vi "Main.vi"(11 "Module Admin":refnum<class "Delacor_lib_QMH_Module Admin.lvclass">) -> ()   [LabVIEW 2024, in "MoneyControl.lvlib"]
doc: "This template is based off of the Queued Message Handler design pattern and the Queued Message Handler project template that ships with LabVIEW.\n\nThe main difference is that the queue is private to this module and communication between modules is performed via Broadcast and Request events.\n\nRequest events are wrapped in public API methods and are handled in the Event Handling Loop (EHL) of this VI. Any module can register for Broadcast events sent by this module. The EHL generates messages based on user interface actions.\n\nThe Message Handling Loop (MHL) processes messages generated by the EHL, or by other messages. The messages are string values, so new messages can be added easily to the Message Cases case structure in the MHL. Each message cluster can also provide an optional value for Message Data, which is a variant that can be converted to whatever message-specific data is required.\n_____\nBased on DQMH Dev Tools: Project Template 7.1.0.1503."
uses:
  MoneyControl.lvlib
  <vilib>/Delacor/Delacor QMH/Libraries/Module Admin_class/Delacor_lib_QMH_Module Admin.lvclass
  Module Data--cluster.ctl
  Stop Argument--cluster.ctl
  <vilib>/Delacor/Delacor QMH/Libraries/Message Queue_class/Delacor_lib_QMH_Message Queue.lvclass/Delacor_lib_QMH_Message Queue.ctl
  <vilib>/Delacor/Delacor QMH/Libraries/Module Admin_class/Delacor_lib_QMH_Module Admin.lvclass/Delacor_lib_QMH_Module Admin.ctl
  Draw FP in Subpanel Argument--cluster.ctl
  Remove From Subpanel Argument--cluster.ctl
  Incrementar Credito Argument--cluster.ctl
  Cancelar Argument--cluster.ctl
  <vilib>/Utility/miscctls.llb/LVFontTypeDef.ctl
  Regresa Cambio Argument--cluster.ctl
  <vilib>/Delacor/Delacor QMH/Libraries/Message Queue_class/Delacor_lib_QMH_Enqueue Message (Single).vi
  <vilib>/Delacor/Delacor QMH/Libraries/Module Admin_class/Delacor_lib_QMH_Get External Launch.vi
  63c2000c-1515-4b81-a1f2-5954ab6849f9.vi
  <vilib>/Delacor/Delacor QMH/Libraries/Message Queue_class/Delacor_lib_QMH_Message Queue.lvclass
  <vilib>/PantherLAB/Message Module/Libraries/Message/PantherLAB_lib_Message.lvlib
panel:
  in  "0.20":bool
  out "Status":string
  in  "1":bool
  in  "0.50":bool
  in  "2":bool
  out "error out":errorcluster
  in  "Cancelar":bool
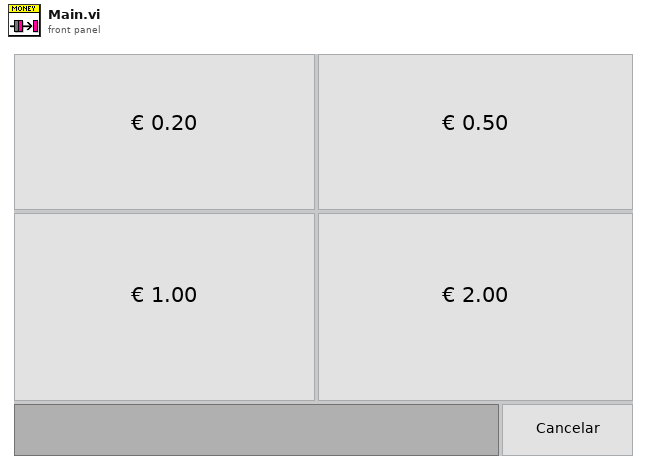
[diagram p1: front panel]
types:
  T1 = typedef "MoneyControl.lvlib/Request Events--cluster.ctl" = cluster{"Stop Module":refnum<user-event>, "Show Panel":refnum<user-event>, "Hide Panel":refnum<user-event>, "Get Module Execution Status":refnum<user-event>, "Show Diagram":refnum<user-event>, "Draw FP in Subpanel":refnum<user-event>, "Remove From Subpanel":refnum<user-event>, "Incrementar Credito":refnum<user-event>, "Cancelar":refnum<user-event>, "Regresa Cambio":refnum<user-event>}
  T2 = typedef "PantherLAB_lib_Message.lvlib/Broadcast Events--cluster.ctl" = cluster{"Module Did Init":refnum<user-event>, "Status Updated":refnum<user-event>, "Error Reported":refnum<user-event>, "Module Did Stop":refnum<user-event>, "Update Module Execution Status":refnum<user-event>}
  T3 = typedef "MoneyControl.lvlib/Module Data--cluster.ctl" = cluster{"Status":string, "Sub Panel":refnum<vi>, "Credito":dbl}
  T4 = enum32{"invalid lock state", "Not Locked", "Locked (No Password)", "Password-protected"}
  T5 = typedef "MoneyControl.lvlib/Stop Argument--cluster.ctl" = cluster{"Origin":string, "Exit via Stop Module Req?":bool, "Wait for Module to stop?":bool}
  T6 = typedef "MoneyControl.lvlib/Draw FP in Subpanel Argument--cluster.ctl" = cluster{"Sub Panel":refnum<vi>}
  T7 = typedef "MoneyControl.lvlib/Remove From Subpanel Argument--cluster.ctl" = cluster{"Boolean":bool}
  T8 = typedef "MoneyControl.lvlib/Incrementar Credito Argument--cluster.ctl" = cluster{"Dinero":dbl}
  T9 = typedef "MoneyControl.lvlib/Cancelar Argument--cluster.ctl" = cluster{"Boolean":bool}
  T10 = typedef "LVFontTypeDef.ctl" = cluster{"Font Name":string, "Size":u16, "Bold":bool, "Italic":bool, "Underline":bool, "Strikeout":bool, "Color":u32}
  T11 = typedef "MoneyControl.lvlib/Regresa Cambio Argument--cluster.ctl" = cluster{"Costo de Producto Vendido":dbl}
  T12 = enum32{"Invalid", "Standard", "Closed", "Hidden", "Minimized", "Maximized"}
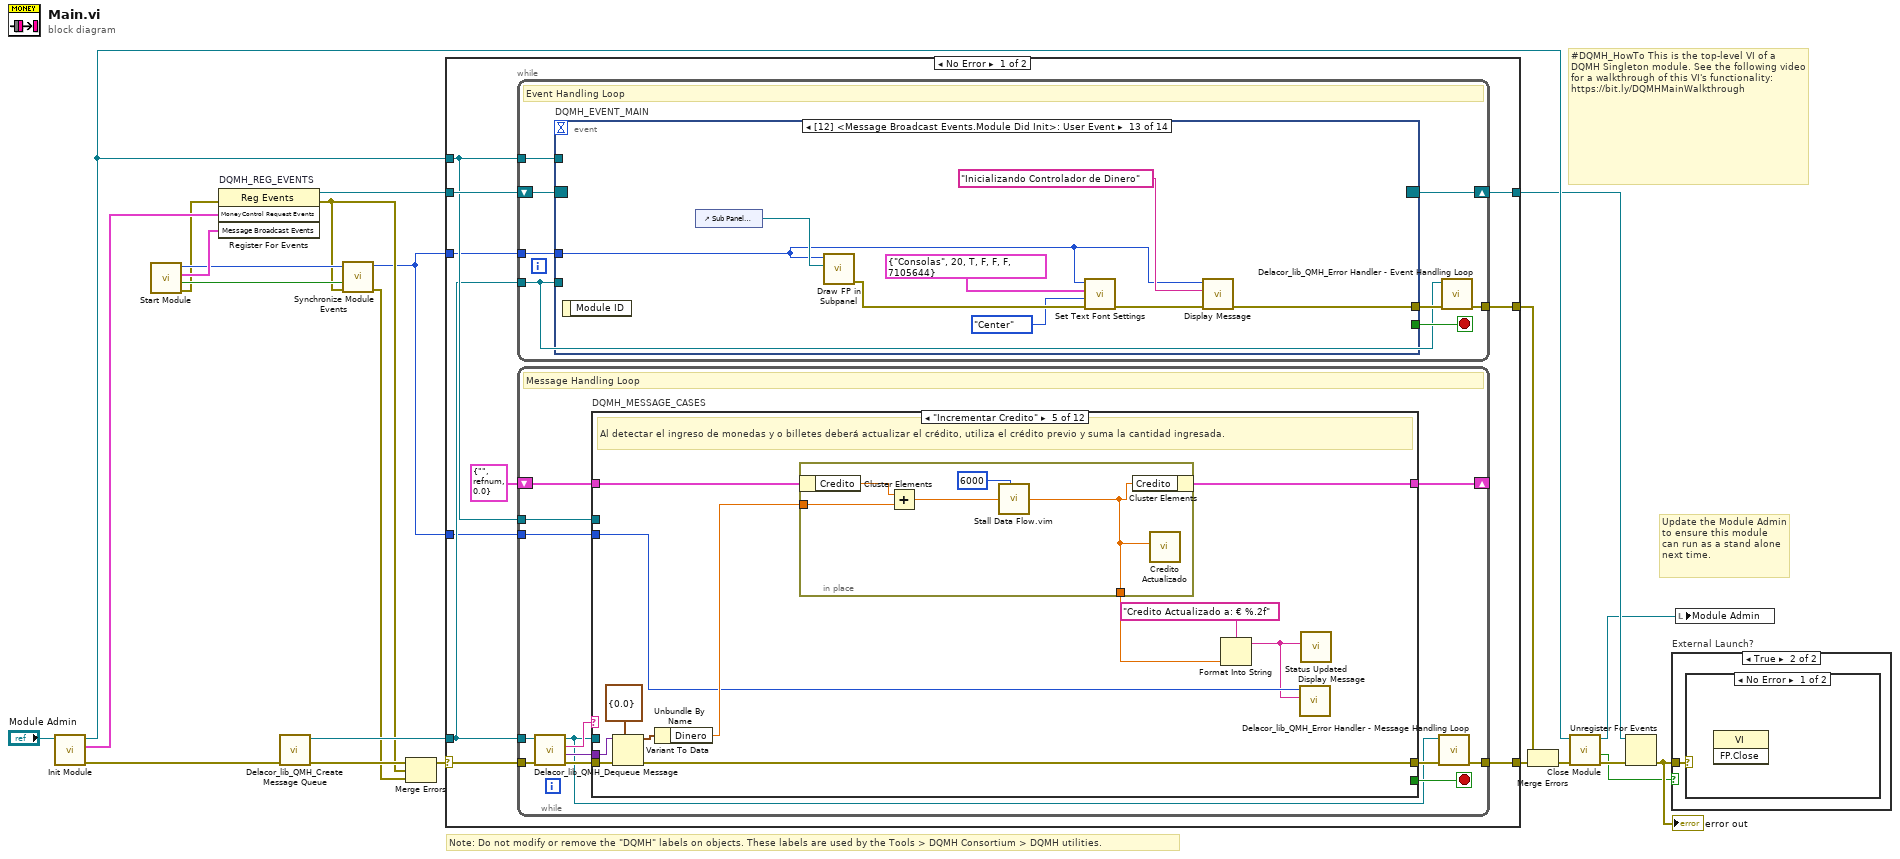
[diagram p0: block diagram]
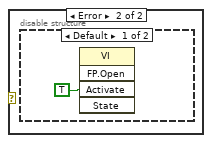
[diagram p3: hidden frame]
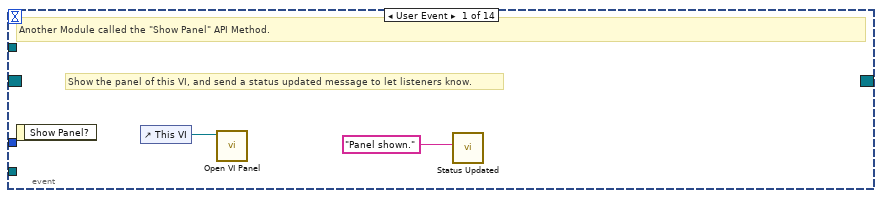
[diagram p5: hidden frame]
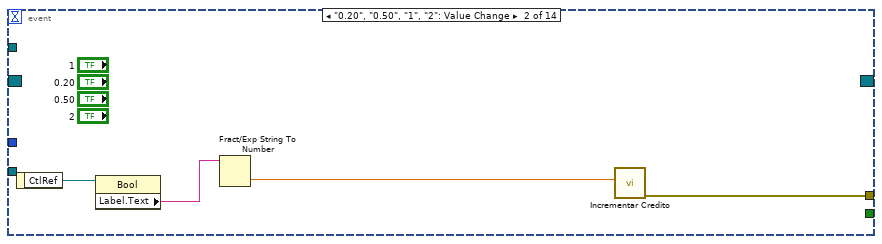
[diagram p6: hidden frame]
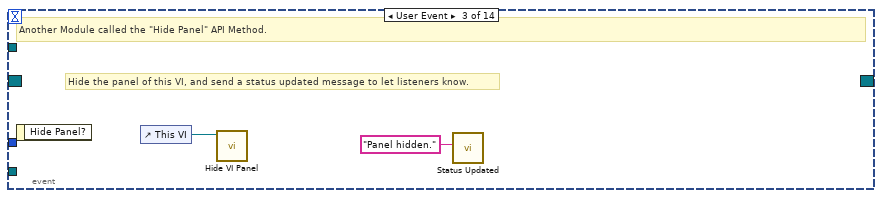
[diagram p7: hidden frame]
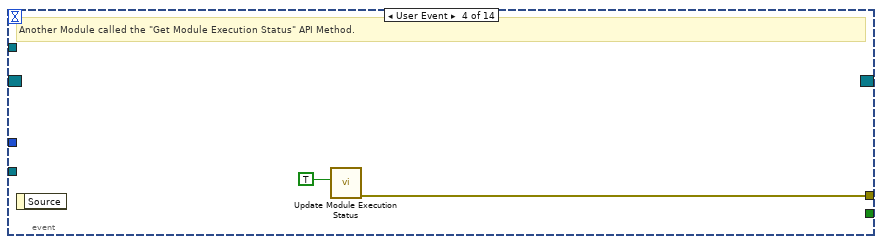
[diagram p8: hidden frame]
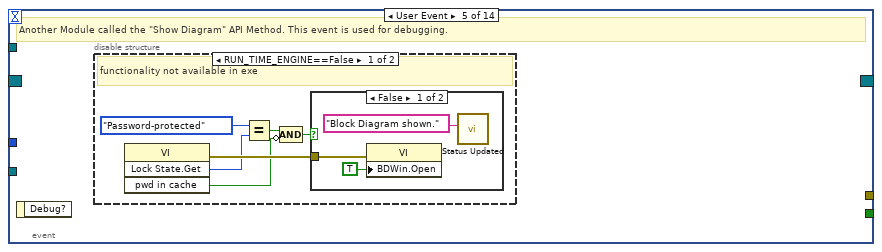
[diagram p9: hidden frame]
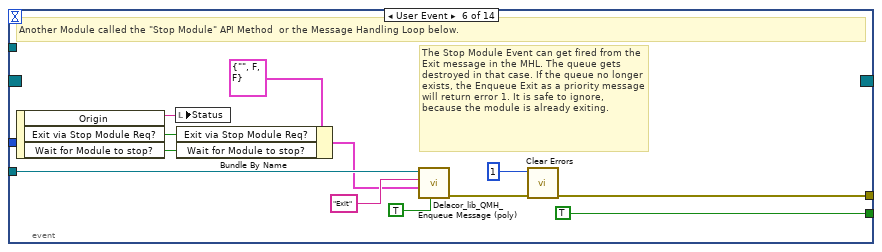
[diagram p12: hidden frame]
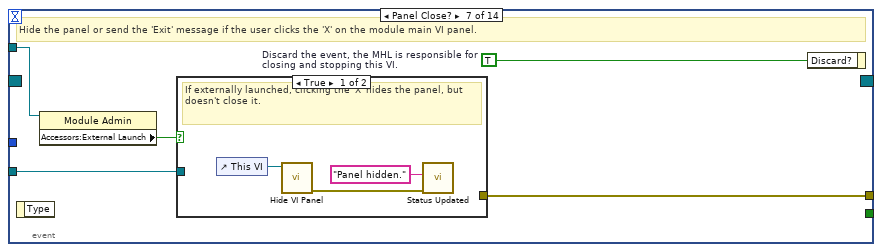
[diagram p13: hidden frame]
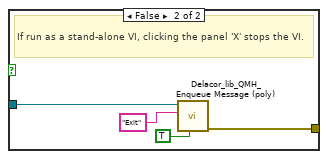
[diagram p14: hidden frame]
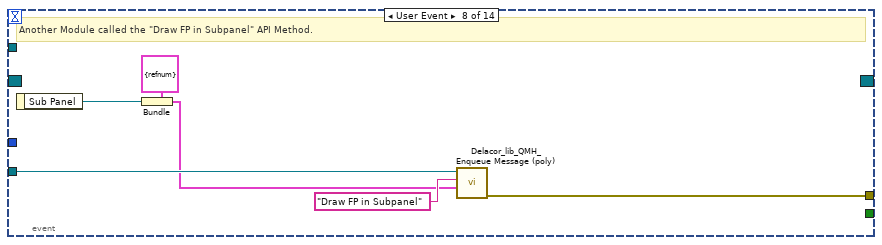
[diagram p15: hidden frame]
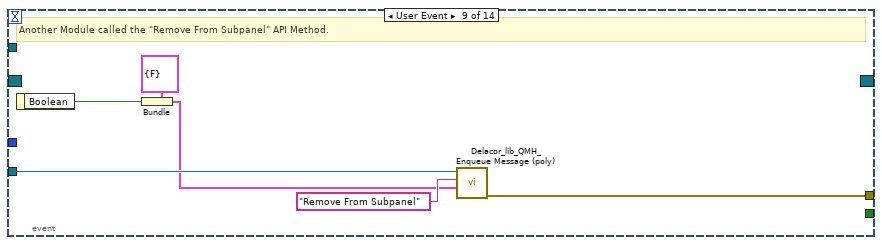
[diagram p16: hidden frame]
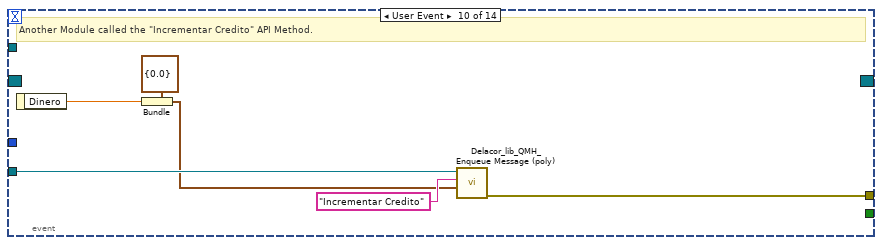
[diagram p17: hidden frame]
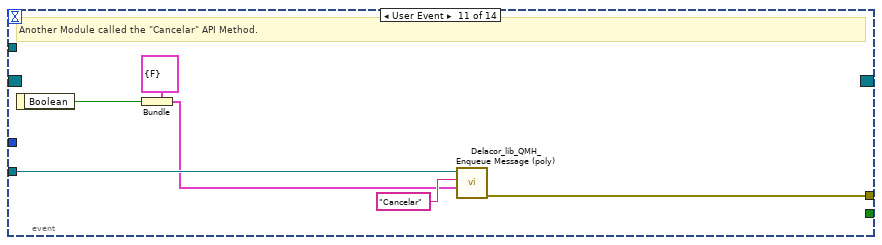
[diagram p18: hidden frame]
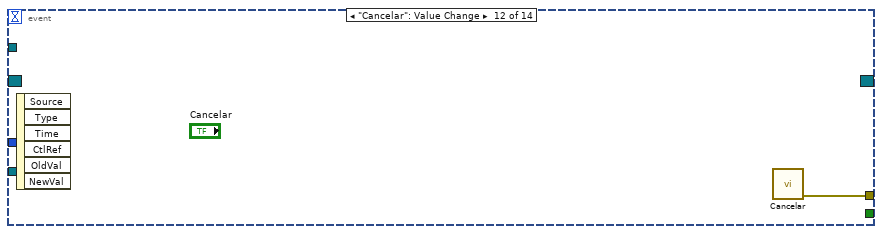
[diagram p19: hidden frame]
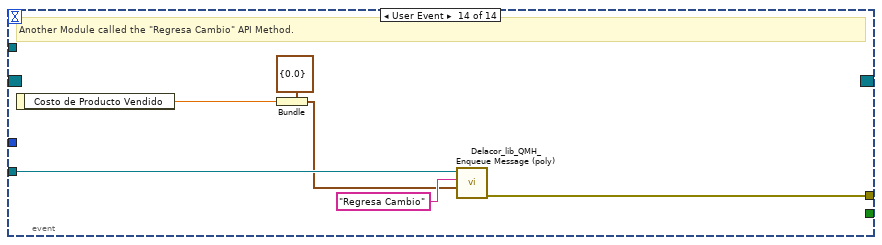
[diagram p20: hidden frame]
diagram:
  # "#DQMH_HowTo This is the top-level VI of a DQMH Singleton module. See the following video for a walkthrough of this VI's functionality: https://bit.ly/DQMHMainWalkthrough"
  # "Note: Do not modify or remove the \"DQMH\" labels on objects. These labels are used by the Tools > DQMH Consortium > DQMH utilities."
  # "Update the Module Admin to ensure this module can run as a stand alone next time."
  n1 = call "Init Module.vi"("Singleton Module Admin in"="Module Admin") -> ("error out"=w22:errorcluster, "MoneyControl Request Events"=w12:T1, "Singleton Module Admin out"=w15:refnum<class "Delacor_lib_QMH_Module Admin.lvclass">)  [unwired: 8 in]
  n2 = call <vilib>:"Start Module.vi"() -> ("error out"=w4:errorcluster, "Wait for Event Sync?"=w5:bool, "Message Broadcast Events"=w7:T2, "Module ID"=w6:i32)  [unwired: 7 in, 1 out]
  n3 = register-events "DQMH_REG_EVENTS"(error in=w4, w12, w7) -> (reference out=w13:refnum<event-registration>, error out=w3:errorcluster)  [unwired: 1 in]
  n4 = call <vilib>:"Delacor_lib_QMH_Create Message Queue.vi"("error in"=w22) -> ("error out"=w17:errorcluster, "Message Queue"=w11:refnum<class "Delacor_lib_QMH_Message Queue.lvclass">)  [unwired: 9 in]
  n5 = call <vilib>:"Synchronize Module Events.vi"("error in"=w3, "Wait for Event Sync?"=w5, "Module ID in"=w6) -> ("error out"=w2:errorcluster, "Module ID out"=w1:i32)  [unwired: 7 in]
  n6 = Merge Errors(w17, w3, w2) -> (w16:errorcluster)
  n7 = case shown="No Error" w16 {
    selector: w16 -> [w31 w304]
    tunnel: [w33 w303] -> w23
    tunnel: [w30 w302] -> w14
    tunnel: w13 -> [w28 w302]
    tunnel: w11 -> [w26 w298]
    tunnel: [w32 _] -> w20
    tunnel: w15 -> [w27 w299]
    tunnel: w1 -> [w25 w296]
    tunnel: w1 -> [w24 _]
    frame No Error {
      n8 = while {
        tunnel: w26 -> [w35]
        shift-right: [w38] -> w30
        shift-left: w28 -> [w39]
        tunnel: [w40] -> w32
        tunnel: w27 -> [w36]
        tunnel: w24 -> [w34]
        stop <- w37 stop-if-true
        # "Event Handling Loop"
        n9 = event "DQMH_EVENT_MAIN" shown="[12] <Message Broadcast Events.Module Did Init>: User Event" {
          selector: w39 -> [_ _ _ _ _ _ _ _ _ _ _ _ _ _]
          dyn-events: [_ _ _ _ _ _ _ _ _ _ _ _ _ _] -> w38
          timeout: _ -> [_ _ _ _ _ _ _ _ _ _ _ _ _ _]
          tunnel: [_ _ _ _ _ TRUE ("Discard?") _ _ _ _ _ _ _ _] -> w37
          tunnel: w35 -> [_ _ _ _ _ w68 w75 w90 w96 w102 w108 _ _ w123]
          tunnel: [_ w45 _ w51 _ w71 w77 w85 w91 w97 w103 w109 w116 w118] -> w41
          tunnel: w36 -> [_ _ _ _ _ _ w74 _ _ _ _ _ _ _]
          tunnel: w34 -> [_ _ _ _ _ _ _ _ _ _ _ _ w112 _]
          event User Event {
            # "Show the panel of this VI, and send a status updated message to let listeners know."
            # "Another Module called the \"Show Panel\" API Method."
            n10 = event-data() -> ()  [unwired: 1 in, 1 out]
            n11 = control-ref of="This VI"() -> (w43:refnum<vi>)
            n12 = call "Open VI Panel.vi"("VI"=w43) -> ()  [unwired: 10 in, 1 out]
            n13 = call "Status Updated.vi"("Status"="Panel shown." ("format string")) -> ()  [unwired: 10 in, 1 out]
          }
          event "0.20", "0.50", "1", "2": Value Change {
            n14 = event-data() -> ("CtlRef"=w47:refnum<vi>)  [unwired: 1 in]
            n15 = property class="Bool"(reference=w47) -> ("Label.Text"=w46:string)  [unwired: 1 in, 2 out]
            n16 = Fract/Exp String To Number(string=w46) -> (number=w44:dbl)  [unwired: 3 in, 1 out]
            n17 = call "Incrementar Credito.vi"("Dinero"=w44) -> ("error out"=w45:errorcluster)  [unwired: 10 in]
          }
          event User Event {
            # "Hide the panel of this VI, and send a status updated message to let listeners know."
            # "Another Module called the \"Hide Panel\" API Method."
            n18 = event-data() -> ()  [unwired: 1 in, 1 out]
            n19 = control-ref of="This VI"() -> (w49:refnum<vi>)
            n20 = call "Hide VI Panel.vi"("VI"=w49) -> ()  [unwired: 10 in, 1 out]
            n21 = call "Status Updated.vi"("Status"="Panel hidden." ("format string")) -> ()  [unwired: 10 in, 1 out]
          }
          event User Event {
            # "Another Module called the \"Get Module Execution Status\" API Method."
            n22 = event-data() -> ()  [unwired: 1 in, 1 out]
            n23 = call "Update Module Execution Status.vi"("Running?"=TRUE) -> ("error out"=w51:errorcluster)  [unwired: 10 in]
          }
          event User Event {
            # "Another Module called the \"Show Diagram\" API Method. This event is used for debugging."
            n24 = event-data() -> ()  [unwired: 1 in, 1 out]
            n25 = disable-structure shown="RUN_TIME_ENGINE==False" {
              frame condition #0 (active) {
                # "functionality not available in exe"
                n26 = invoke on="Invoke Node" class="VI" method="Lock State.Get"() -> (error out=w57:errorcluster, "Get Lock State"=w56:T4, "pwd in cache"=w53:bool)  [unwired: 4 in, 1 out]
                n27 = Equal?(x=T4."Password-protected", y=w56) -> (x = y?=w54:bool)
                n28 = Compound Arithmetic op=AND(w54, invert w53) -> (w52:bool)
                n29 = case shown="False" w52 {
                  tunnel: w57 -> [w60 _]
                  frame False {
                    n30 = property on="Property Node" class="VI"(error in=w60, "BDWin.Open"=TRUE ("Block Diagram Window:Open")) -> ()  [unwired: 1 in, 2 out]
                    n31 = call "Status Updated.vi"("Status"="Block Diagram shown." ("format string")) -> ()  [unwired: 10 in, 1 out]
                  }
                  frame True {
                    # "Password-protected VI, and the password is not in the cache. Do not show the diagram."
                  }
                }
              }
              frame condition #1 {
              }
            }
          }
          event User Event {
            # "The Stop Module Event can get fired from the Exit message in the MHL. The queue gets destroyed in that case. If the queue no longer exists, the Enqueue Exit as a priority message will return error 1. It is safe to ignore, because the module is already exiting."
            # "Another Module called the \"Stop Module\" API Method  or the Message Handling Loop below."
            n32 = event-data() -> ("Origin"=w67:string, "Exit via Stop Module Req?"=w63:bool, "Wait for Module to stop?"=w62:bool)  [unwired: 1 in]
            n33 = local write "Status"(w67) -> ()
            n34 = Bundle By Name(cluster=T5 {"Origin"="", "Exit via Stop Module Req?"=FALSE, "Wait for Module to stop?"=FALSE} ("Stop Argument"), "Exit via Stop Module Req?"=w63, "Wait for Module to stop?"=w62) -> (w61:T5)
            n35 = call-poly <vilib>:"Delacor_lib_QMH_Enqueue Message (poly).vi"("Priority Message? (F)"=TRUE, "Message Data"=w61, "Message"="Exit", "Message Queue in"=w68) -> ("error out"=w72:errorcluster)  [unwired: 6 in, 1 out]
            n36 = call <vilib>:"Clear Errors.vi"("error in (no error)"=w72, "specific error code to clear (0: all)"=1) -> ("error out"=w71:errorcluster)  [unwired: 4 in, 1 out]
          }
          event Panel Close? {
            w76 = TRUE  # Discard the event, the MHL is responsible for closing and stopping this VI.
            # "Hide the panel or send the 'Exit' message if the user clicks the 'X' on the module main VI panel."
            n37 = event-data() -> ()  [unwired: 1 in, 1 out]
            n38 = property on="Property Node" class="Module Admin"(reference=w74) -> ("Accessors:External Launch"=w73:bool)  [unwired: 1 in, 2 out]
            n39 = case shown="True" w73 {
              tunnel: w75 -> [_ w83]
              tunnel: [_ w84] -> w77
              frame True {
                # "If externally launched, clicking the 'X' hides the panel, but doesn't close it."
                n40 = control-ref of="This VI"() -> (w80:refnum<vi>)
                n41 = call "Hide VI Panel.vi"("VI"=w80) -> ("error out"=w78:errorcluster)  [unwired: 10 in]
                n42 = call "Status Updated.vi"("error in"=w78, "Status"="Panel hidden." ("format string")) -> ()  [unwired: 9 in, 1 out]
              }
              frame False {
                # "If run as a stand-alone VI, clicking the panel 'X' stops the VI."
                n43 = call-poly <vilib>:"Delacor_lib_QMH_Enqueue Message (poly).vi"("Priority Message? (F)"=TRUE, "Message"="Exit", "Message Queue in"=w83) -> ("error out"=w84:errorcluster)  [unwired: 7 in, 1 out]
              }
            }
            n44 = event-data ("Event Filter Node")("Discard?"=w76) -> ()  [unwired: 1 in, 1 out]
          }
          event User Event {
            # "Another Module called the \"Draw FP in Subpanel\" API Method."
            n45 = event-data() -> ("Sub Panel"=w86:refnum<vi>)  [unwired: 1 in]
            n46 = Bundle(cluster=T6 {"Sub Panel"=refnum} ("Draw FP in Subpanel Argument"), "Sub Panel"=w86) -> (w87:T6)
            n47 = call-poly <vilib>:"Delacor_lib_QMH_Enqueue Message (poly).vi"("Message Data"=w87, "Message"="Draw FP in Subpanel", "Message Queue in"=w90) -> ("error out"=w85:errorcluster)  [unwired: 7 in, 1 out]
          }
          event User Event {
            # "Another Module called the \"Remove From Subpanel\" API Method."
            n48 = event-data() -> ("Boolean"=w92:bool)  [unwired: 1 in]
            n49 = Bundle(cluster=T7 {"Boolean"=FALSE} ("Remove From Subpanel Argument"), "Boolean"=w92) -> (w93:T7)
            n50 = call-poly <vilib>:"Delacor_lib_QMH_Enqueue Message (poly).vi"("Message Data"=w93, "Message"="Remove From Subpanel", "Message Queue in"=w96) -> ("error out"=w91:errorcluster)  [unwired: 7 in, 1 out]
          }
          event User Event {
            # "Another Module called the \"Incrementar Credito\" API Method."
            n51 = event-data() -> ("Dinero"=w98:dbl)  [unwired: 1 in]
            n52 = Bundle(cluster=T8 {"Dinero"=0.0} ("Incrementar Credito Argument"), "Dinero"=w98) -> (w99:T8)
            n53 = call-poly <vilib>:"Delacor_lib_QMH_Enqueue Message (poly).vi"("Message Data"=w99, "Message"="Incrementar Credito", "Message Queue in"=w102) -> ("error out"=w97:errorcluster)  [unwired: 7 in, 1 out]
          }
          event User Event {
            # "Another Module called the \"Cancelar\" API Method."
            n54 = event-data() -> ("Boolean"=w104:bool)  [unwired: 1 in]
            n55 = Bundle(cluster=T9 {"Boolean"=FALSE} ("Cancelar Argument"), "Boolean"=w104) -> (w105:T9)
            n56 = call-poly <vilib>:"Delacor_lib_QMH_Enqueue Message (poly).vi"("Message Data"=w105, "Message"="Cancelar", "Message Queue in"=w108) -> ("error out"=w103:errorcluster)  [unwired: 7 in, 1 out]
          }
          event "Cancelar": Value Change {
            n57 = event-data() -> ()  [unwired: 1 in, 6 out]
            n58 = call "Cancelar.vi"() -> ("error out"=w109:errorcluster)  [unwired: 11 in]
          }
          event User Event {
            n59 = event-data() -> ()  [unwired: 1 in, 1 out]
            n60 = control-ref of="Sub Panel Mensajes"() -> (w117:refnum<vi>)
            n61 = call <vilib>:"Draw FP in Subpanel.vi"("Sub Panel"=w117, "Module ID"=w112) -> ("error out"=w114:errorcluster)  [unwired: 9 in]
            n62 = call <vilib>:"Set Text Font Settings.vi"("error in"=w114, "Text.Justification"=enum16{"Left", "Center", "Right"}."Center", "Font"=T10 {"Font Name"="Consolas", "Size"=20, "Bold"=TRUE, "Italic"=FALSE, "Underline"=FALSE, "Strikeout"=FALSE, "Color"=7105644}, "Module ID"=w112) -> ("error out"=w113:errorcluster)  [unwired: 7 in]
            n63 = call <vilib>:"Display Message.vi"("error in"=w113, "Message"="Inicializando Controlador de Dinero", "Module ID"=w112) -> ("error out"=w116:errorcluster)  [unwired: 8 in]
          }
          event User Event {
            # "Another Module called the \"Regresa Cambio\" API Method."
            n64 = event-data() -> ("Costo de Producto Vendido"=w119:dbl)  [unwired: 1 in]
            n65 = Bundle(cluster=T11 {"Costo de Producto Vendido"=0.0} ("Regresa Cambio Argument"), "Costo de Producto Vendido"=w119) -> (w120:T11)
            n66 = call-poly <vilib>:"Delacor_lib_QMH_Enqueue Message (poly).vi"("Message Data"=w120, "Message"="Regresa Cambio", "Message Queue in"=w123) -> ("error out"=w118:errorcluster)  [unwired: 7 in, 1 out]
          }
        }
        n67 = call-dynamic "Delacor_lib_QMH_Error Handler - Event Handling Loop.vi"("error in"=w41, "Message Queue in"=w35) -> ("dup error in"=w40:errorcluster)  [unwired: 8 in, 1 out]
      }
      n68 = while {
        tunnel: w26 -> [w125]
        shift-right: [w133] -> _
        shift-left: T3 {"Status"="", "Sub Panel"=refnum, "Credito"=0.0} ("Data Cluster") -> [w134]
        tunnel: w31 -> [w136]
        tunnel: [w128] -> w33
        tunnel: w27 -> [w129]
        tunnel: w25 -> [w124]
        stop <- w132 stop-if-true
        # "Message Handling Loop"
        n69 = call-dynamic "Delacor_lib_QMH_Dequeue Message.vi"("error in"=w136, "Message Queue in"=w125) -> ("error out"=w135:errorcluster, "Message Data"=w130:variant, "Message"=w131:string, "Message Queue out"=w126:refnum<class "Delacor_lib_QMH_Message Queue.lvclass">)  [unwired: 6 in]
        n70 = case "DQMH_MESSAGE_CASES" shown="\"Incrementar Credito\"" w131 {
          selector: w131 -> [_ _ _ _ _ _ _ _ _ _ _ w291]
          tunnel: w126 -> [_ _ _ _ _ _ _ _ _ w253 w279 _]
          tunnel: w135 -> [w154 w158 w174 w192 w210 w223 w237 w247 w249 w260 w285 w294]
          tunnel: [w152 w158 w166 w186 w209 w222 w236 w246 w249 w256 w280 w295] -> w127
          tunnel: w134 -> [w143 w157 w173 w188 w203 w218 w232 w245 w248 w255 w271 w292]
          tunnel: [w142 w157 w169 w183 w204 w217 w230 w245 w248 w255 w271 w292] -> w133
          tunnel: [_ _ _ _ _ _ _ _ _ _ w278 _] -> w132
          tunnel: w130 -> [_ _ w172 w191 w208 w221 w235 _ _ w254 w277 _]
          tunnel: w129 -> [w144 _ _ _ _ _ _ _ _ w252 w272 _]
          tunnel: w124 -> [_ _ _ _ w200 w216 w229 _ _ _ w269 _]
          frame "Initialize" {
            w138 = "Initial Message" ("Initial Message")
            # "#DQMH_CodeNeeded - Initialize the appearance of the front panel."
            # "#DQMH_CodeNeeded - Initialize your state data here."
            # "Initialize - Any operation that needs to be done before the module can receive messages. Synchronize Caller Events.vi will inform Start Module.vi that the module has launched and is ready to receive messages. Module Did Init.vi will broadcast that the module initialized."
            n71 = call "Synchronize Caller Events.vi"("error in"=w154, "Singleton Module Admin in"=w144) -> ("error out"=w153:errorcluster, "Singleton Module Admin out"=w139:refnum<class "Delacor_lib_QMH_Module Admin.lvclass">)  [unwired: 8 in]
            n72 = property on="Property Node" class="Module Admin"(reference=w139) -> ("Accessors:External Launch"=w148:bool)  [unwired: 1 in, 2 out]
            n73 = Select(t=T12."Hidden" ("State"), s=w148, f=T12."Standard" ("State")) -> (s? t:f=w145:T12)
            n74 = call "Module Name--constant.vi"() -> ("Module Name"=w151:string)  [unwired: 11 in]
            n75 = property on="Property Node" class="VI"("Front Panel.Title"=w151) -> (reference out=w150:refnum<vi>, error out=w156:errorcluster)  [unwired: 2 in]
            n76 = invoke on="Invoke Node" class="VI" method="FP.Open"(reference=w150, error in=w156, "State"=w145) -> (reference out=w149:refnum<vi>, error out=w155:errorcluster)  [unwired: 2 in, 3 out]
            n77 = Bundle By Name(cluster=w143, "Status"=w138) -> (w142:T3)
            n78 = invoke on="Invoke Node" class="VI" method="FP.Center"(reference=w149, error in=w155) -> ()  [unwired: 1 in, 3 out]
            n79 = call "Credito Actualizado.vi"("Credito"=0.0) -> ()  [unwired: 10 in, 1 out]
            n80 = call "Module Name--constant.vi"() -> ("Module Name"=w140:string)  [unwired: 11 in]
            n81 = call "Module Did Init.vi"("error in"=w153, "Initialized?"=TRUE, "Origin"=w140) -> ("error out"=w152:errorcluster)  [unwired: 8 in]
            "Status" <- w138
          }
          frame "---Module Specific---" {
            # "Separator -- The following cases handle messages specific to this Module."
          }
          frame "Draw FP in Subpanel" {
            # "Draw FP in Subpanel"
            n82 = Variant To Data(error in=w174, type=T6 {"Sub Panel"=refnum} ("Draw FP in Subpanel Argument"), Variant=w172) -> (data=w170:T6, error out=w164:errorcluster)
            n83 = Unbundle By Name(w170) -> ("Sub Panel"=w168:refnum<vi>)
            n84 = control-ref of="This VI"() -> (w161:refnum<vi>)
            n85 = property class="VI"(reference=w161, error in=w164) -> (reference out=w160:refnum<vi>, error out=w162:errorcluster, "FP.State"=w159:T12)
            n86 = case shown="\"Closed\"" w159 {
              tunnel: [w176 w180] -> w165
              tunnel: [w175 w179] -> w163
              tunnel: w162 -> [w175 w178]
              tunnel: w160 -> [w176 w177]
              frame "Closed" {
              }
              frame "Standard", Default {
                n87 = invoke class="VI" method="FP.Close"(reference=w177, error in=w178) -> (reference out=w180:refnum<vi>, error out=w179:errorcluster)  [unwired: 1 in, 1 out]
              }
            }
            n88 = invoke class="SubPnl" method="Insert VI"(reference=w168, error in=w163, "VI Ref"=w165) -> (reference out=w167:refnum<vi>, error out=w166:errorcluster)  [unwired: 1 in, 2 out]
            n89 = Bundle By Name(cluster=w173, "Sub Panel"=w167) -> (w169:T3)
          }
          frame "Remove From Subpanel" {
            # "Remove From Subpanel"
            n90 = Variant To Data(error in=w192, type=T7 {"Boolean"=FALSE} ("Remove From Subpanel Argument"), Variant=w191) -> (data=w189:T7, error out=w187:errorcluster)
            n91 = Unbundle By Name(w189) -> ()  [unwired: 1 out]
            n92 = Unbundle By Name(w188) -> ("Sub Panel"=w185:refnum<vi>)
            n93 = Not A Number/Path/Refnum?(number/path/refnum=w185) -> (NaN/Path/Refnum?=w184:bool)
            n94 = case shown="True" w184 {
              tunnel: w187 -> [w196 w198]
              tunnel: [w195 w198] -> w186
              tunnel: w185 -> [w194 _]
              tunnel: ["Module Removed from Subpanel" "This module has not been inserted into the subpanel"] -> w181
              frame False {
                n95 = invoke class="SubPnl" method="Remove VI"(reference=w194, error in=w196) -> (error out=w195:errorcluster)  [unwired: 1 in, 2 out]
              }
              frame True {
              }
            }
            n96 = Bundle By Name(cluster=w188, "Sub Panel"=refnum<vi> refnum) -> (w183:T3)
            n97 = call "Status Updated.vi"("Status"=w181) -> ()  [unwired: 10 in, 1 out]
          }
          frame "Incrementar Credito" {
            # "Al detectar el ingreso de monedas y o billetes deberá actualizar el crédito, utiliza el crédito previo y suma la cantidad ingresada."
            n98 = Variant To Data(error in=w210, type=T8 {"Dinero"=0.0} ("Incrementar Credito Argument"), Variant=w208) -> (data=w206:T8, error out=w209:errorcluster)
            n99 = Unbundle By Name(w206) -> ("Dinero"=w205:dbl)
            n100 = in-place {
              in-place-border: w205 -> [w214]
              in-place-border: [w212] -> w202
              n101 = in-place-cluster #1(w203) -> ("Credito"=w215:dbl)
              n102 = Add(x=w215, y=w214) -> (x+y=w213:dbl)
              n103 = call "Stall Data Flow.vim"("value in"=w213, "milliseconds to wait"=u32 6000) -> ("value out"=w212:dbl)  [unwired: 1 out]
              n104 = in-place-cluster #1("Credito"=w212) -> (w204:T3)
              n105 = call "Credito Actualizado.vi"("Credito"=w212) -> ()  [unwired: 10 in, 1 out]
            }
            n106 = Format Into String(format string="Credito Actualizado a: € %.2f", w202) -> (resulting string=w199:string)  [unwired: 2 in, 1 out]
            n107 = call <vilib>:"Display Message.vi"("Message"=w199, "Module ID"=w200) -> ()  [unwired: 9 in, 1 out]
            n108 = call "Status Updated.vi"("Status"=w199) -> ()  [unwired: 10 in, 1 out]
          }
          frame "Cancelar" {
            # "Regresa la totalidad del crédito actual"
            n109 = Variant To Data(error in=w223, type=T9 {"Boolean"=FALSE} ("Cancelar Argument"), Variant=w221) -> (data=w219:T9, error out=w222:errorcluster)
            n110 = Unbundle By Name(w219) -> ()  [unwired: 1 out]
            n111 = in-place {
              in-place-border: w216 -> [w226]
              w224 = 0.0 ("Credito")
              n112 = in-place-cluster #2(w218) -> ("Credito"=w228:dbl)
              n113 = Format Into String(format string="Operacion Cancelada por el Usuario Regresando Credito: € %.2f", w228) -> (resulting string=w225:string)  [unwired: 2 in, 1 out]
              n114 = call "Status Updated.vi"("Status"=w225) -> ()  [unwired: 10 in, 1 out]
              n115 = call <vilib>:"Display Message.vi"("Message"=w225, "Module ID"=w226) -> ()  [unwired: 9 in, 1 out]
              n116 = in-place-cluster #2("Credito"=w224) -> (w217:T3)
              n117 = call "Credito Actualizado.vi"("Credito"=w224) -> ()  [unwired: 10 in, 1 out]
            }
          }
          frame "Regresa Cambio" {
            # "Request para regresar cambio, cuando se hace la venta de productos, realiza la resta del credito menos el costo del producto"
            n118 = Variant To Data(error in=w237, type=T11 {"Costo de Producto Vendido"=0.0} ("Regresa Cambio Argument"), Variant=w235) -> (data=w233:T11, error out=w236:errorcluster)
            n119 = Unbundle By Name(w233) -> ("Costo de Producto Vendido"=w231:dbl)
            n120 = in-place {
              in-place-border: w231 -> [w243]
              in-place-border: w229 -> [w242]
              w238 = 0.0 ("Credito")
              n121 = in-place-cluster #3(w232) -> ("Credito"=w244:dbl)
              n122 = Subtract(x=w244, y=w243) -> (x-y=w241:dbl)
              n123 = Format Into String(format string="Recoje tu Cambio: € %.2f, Credito Actual: € %.2f", w241, w238) -> (resulting string=w240:string)  [unwired: 2 in, 1 out]
              n124 = call <vilib>:"Display Message.vi"("Message"=w240, "Module ID"=w242) -> ()  [unwired: 9 in, 1 out]
              n125 = call "Credito Actualizado.vi"("Credito"=w238) -> ()  [unwired: 10 in, 1 out]
              n126 = in-place-cluster #3("Credito"=w238) -> (w230:T3)
            }
          }
          frame "---Copy This Frame---" {
            # "Duplicate this frame when creating new messages.  Change this comment in the duplicated frame to describe this message."
            n127 = Merge Errors(w247) -> (w246:errorcluster)
          }
          frame "---Exit and Error Handling---" {
            # "Separator - The following cases handle errors and exit messages."
          }
          frame "Error" {
            # "#DQMH_CodeRecommended - If the module is running in standalone mode (External Launch = FALSE), this code will pop up an error dialog and call the 'Exit' message if an error occurs. Add more fine-grained error management here."
            # "Error - Check the error message data and respond accordingly. This message is sent by the \"Error Handler\" VIs at the end of each loop in this application."
            n128 = property on="Property Node" class="Module Admin"(reference=w252) -> ("Accessors:External Launch"=w251:bool)  [unwired: 1 in, 2 out]
            n129 = Variant To Data(error in=w260, type=errorcluster {"status"=FALSE, "code"=0, "source"=""} ("error constant"), Variant=w254) -> (data=w250:errorcluster, error out=w258:errorcluster)
            n130 = local write "error out"(w250) -> ()
            n131 = call "Error Reported.vi"("Error"=w250) -> ()  [unwired: 10 in, 1 out]
            n132 = case shown="False" w251 {
              tunnel: [w265 _] -> w257
              tunnel: w253 -> [w263 _]
              tunnel: w250 -> [w264 _]
              frame False {
                n133 = disable-structure shown="Default" {
                  disable-tunnel: w264 -> [w266 _]
                  frame condition #0 (active) {
                    # "If the module is running standalone, then pop up an error dialog and call the \"Exit\" message."
                    n134 = call <vilib>:"Simple Error Handler.vi"("error in (no error)"=w266) -> ()  [unwired: 4 in, 5 out]
                  }
                  frame condition #1 {
                    # "To prevent the Simple Error Handler VI from being loaded (e.g. when deploying to a Real-Time target), add the Conditional Disable Symbol \"DQMH_Disable_SEH\" to your project and set it to TRUE."
                  }
                }
                n135 = call-poly <vilib>:"Delacor_lib_QMH_Enqueue Message (poly).vi"("Priority Message? (F)"=TRUE, "Message"="Exit", "Message Queue in"=w263) -> ("error out"=w265:errorcluster)  [unwired: 7 in, 1 out]
              }
              frame True {
                # "If the module was launched externally, calling the Error Reported broadcast VI is the only action performed by the \"Error\" message. The module's caller can then process the error appropriately."
              }
            }
            n136 = Merge Errors(w258, w257) -> (w256:errorcluster)
          }
          frame "Exit" {
            w276 = 91  # 91: not all Exit messages will have an argument
            w278 = TRUE  # Stop the VI
            # "Release the message queue reference"
            # "Exit - Exit the application."
            n137 = Variant To Data(error in=w285, type=T5 {"Origin"="", "Exit via Stop Module Req?"=FALSE, "Wait for Module to stop?"=FALSE} ("Stop Argument"), Variant=w277) -> (data=w274:T5, error out=w282:errorcluster)
            n138 = call <vilib>:"Clear Errors.vi"("error in (no error)"=w282, "specific error code to clear (0: all)"=w276) -> ("error out"=w284:errorcluster)  [unwired: 4 in, 1 out]
            n139 = control-ref of="This VI"() -> (w273:refnum<vi>)
            n140 = call-dynamic "Delacor_lib_QMH_Release Message Queue.vi"("error in"=w284, "Message Queue"=w279) -> ("error out"=w283:errorcluster)  [unwired: 9 in]
            n141 = call "Handle Exit.vi"("Stop Argument"=w274, "Admin in"=w272, "VI reference"=w273) -> ("error out"=w281:errorcluster)  [unwired: 7 in, 1 out]
            n142 = Unbundle By Name(w271) -> ("Sub Panel"=w270:refnum<vi>)
            n143 = invoke class="SubPnl" method="Remove VI"(reference=w270) -> ()  [unwired: 2 in, 3 out]
            n144 = call <vilib>:"Stop Module.vi"("Origin"="MoneyControl Sent Stop", "Module ID"=w269) -> ("error out"=w267:errorcluster)  [unwired: 9 in]
            n145 = Merge Errors(w283, w281, w267) -> (w280:errorcluster)
            n146 = call "Error Reported.vi"("Error"=w280) -> ()  [unwired: 10 in, 1 out]
          }
          frame Default {
            # "'Default' case only runs if there is a message that isn't defined in any of the other cases.  Output a programming error."
            n147 = call "Module Name--constant.vi"() -> ("Module Name"=w290:string)  [unwired: 11 in]
            n148 = Format Into String(format string="The invalid message string \"%s\" was received in the Message Handling Loop for module \"%s\".", w291, w290) -> (resulting string=w286:string)  [unwired: 2 in, 1 out]
            n149 = call <vilib>:"Error Cluster From Error Code.vi"("show call chain? (False)"=TRUE, "error message (\"\")"=w286, "error code (0)"=1) -> ("error out"=w293:errorcluster)  [unwired: 6 in]
            n150 = Merge Errors(w294, w293) -> (w295:errorcluster)
          }
        }
        n151 = call-dynamic "Delacor_lib_QMH_Error Handler - Message Handling Loop.vi"("error in"=w127, "Message Queue in"=w126) -> ("dup error in"=w128:errorcluster)  [unwired: 8 in, 1 out]
      }
    }
    frame Error {
      # "Synchronize Caller Events.vi will inform Start Module.vi that the module has launched and will let the code calling Start Module.vi register for broadcasts and would permit the caller receive the broadcast that an error occurred at launch time."
      n152 = call-dynamic "Delacor_lib_QMH_Release Message Queue.vi"("error in"=w304, "Message Queue"=w298) -> ("error out"=w303:errorcluster)  [unwired: 9 in]
      n153 = call "Synchronize Caller Events.vi"("Singleton Module Admin in"=w299) -> ("error out"=w305:errorcluster)  [unwired: 9 in, 1 out]
      n154 = call "Module Name--constant.vi"() -> ("Module Name"=w301:string)  [unwired: 11 in]
      n155 = Format Into String(format string="An error occurred during initialization. %s is no longer running.", w301) -> (resulting string=w297:string)  [unwired: 2 in, 1 out]
      n156 = Merge Errors(w303, w305) -> (w306:errorcluster)
      n157 = call "Error Reported.vi"("Additional Information"=w297, "Error"=w306) -> ()  [unwired: 9 in, 1 out]
      n158 = call <vilib>:"Stop Module.vi"("Origin"=w297, "Module ID"=w296) -> ()  [unwired: 9 in, 1 out]
    }
  }
  n159 = Merge Errors(w20, w23) -> (w19:errorcluster)
  n160 = call "Close Module.vi"("error in"=w19, "Module Admin in"=w15) -> ("error out"=w21:errorcluster, "External Launch"=w8:bool, "Module Admin out"=w9:refnum<class "Delacor_lib_QMH_Module Admin.lvclass">)  [unwired: 7 in]
  n161 = Unregister For Events(event registration refnum=w14, error in=w21) -> (error out=w18:errorcluster)
  "error out" <- w18
  n162 = case "External Launch?" shown="True" w8 {
    tunnel: w18 -> [_ w307]
    frame False {
    }
    frame True {
      n163 = case shown="No Error" w307 {
        frame No Error {
          n164 = invoke on="Invoke Node" class="VI" method="FP.Close"() -> ()  [unwired: 3 in, 3 out]
        }
        frame Error {
          n165 = disable-structure shown="Default" {
            frame condition #0 (active) {
              n166 = invoke class="VI" method="FP.Open"("Activate"=TRUE ("Activate?")) -> ()  [unwired: 4 in, 5 out]
            }
            frame condition #1 {
              # "Don't show panel on error if running inside a built EXE."
            }
          }
        }
      }
    }
  }
  n167 = local write "Module Admin"(w9) -> ()
